vi "Res_stabiliz.vi"(4 "Точность ThRes":dbl step=0.01, 5 "Up_Volt_limit":dbl=5.0, 6 "Optimum ThRes":dbl format="%#_6f", 7 "Low_Volt_limit":dbl=1.0, 8 "TEC_Source":refnum<k15> caption="instrument handle", 9 "4070_address":refnum<k15>="PXI3Slot6_4 (1)" caption="4070_out", 10 "channel name":string, 11 "Start Voltage":dbl=3.0 format="%#.7f") -> (0 "Error message":string, 1 "Подстроенное напряжение":dbl, 2 "ThRes value":dbl, 3 "thRes_adj":dbl format="%0.2f")   [LabVIEW 2013]
uses:
  <instrlib>/niDMM/nidmm.llb/niDMM Resolution in Digits.ctl
  <instrlib>/niDMM/nidmm.llb/niDMM Function.ctl
  <vilib>/Analysis/baseanly.llb/Mean (DBL).vi
  <instrlib>/niDMM/nidmm.llb/niDMM Configure Measurement Digits.vi
  <vilib>/Analysis/NI_AALBase.lvlib
panel:
  out "Необходимая подстройка\nНапряжения":dbl
  out "Разница ThRes":dbl
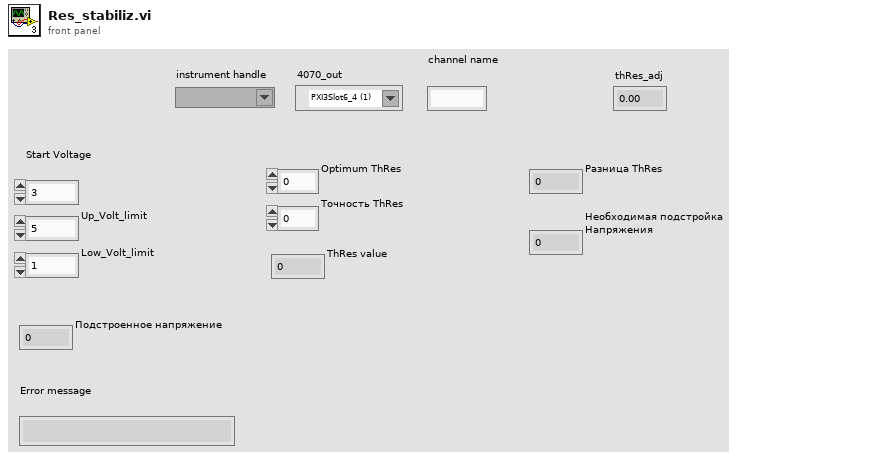
[diagram p1: front panel]
types:
  T1 = typedef "niDMM Function.ctl" = enum16{"DC Volts", "AC Volts", "DC Current", "AC Current", "2-wire Resistance", "4-wire Resistance", "Diode", "Frequency", "Period", "AC Volts DC Coupled", "Capacitance", "Inductance", "Temperature"}
  T2 = typedef "niDMM Resolution in Digits.ctl" = dbl
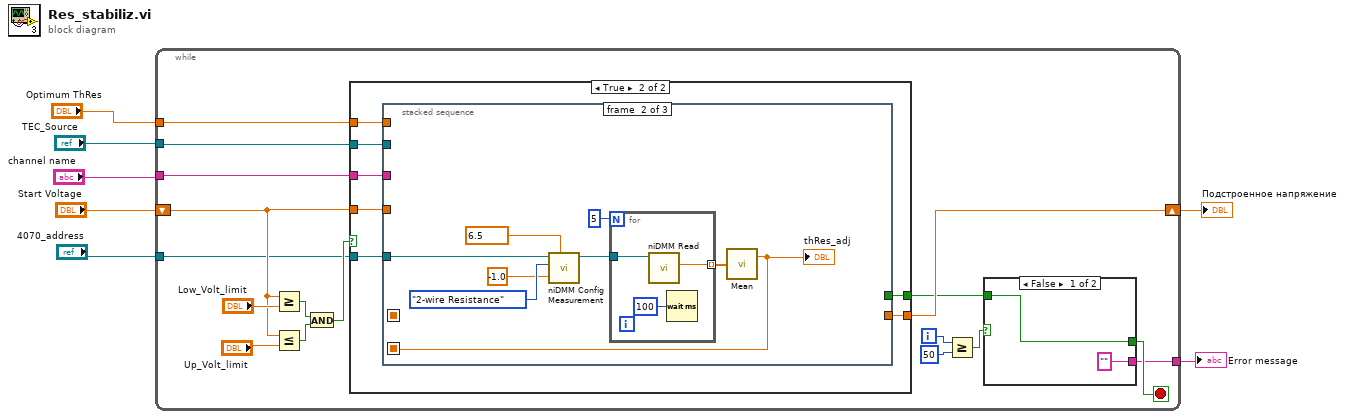
[diagram p0: block diagram]
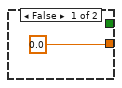
[diagram p2: hidden frame]
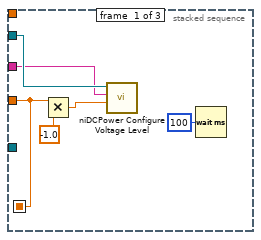
[diagram p3: hidden frame]
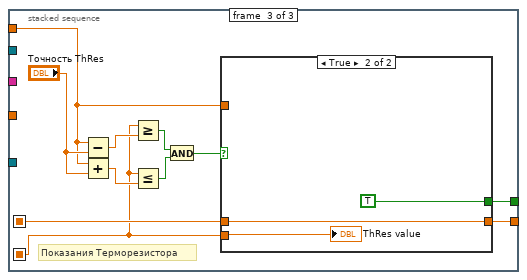
[diagram p4: hidden frame]
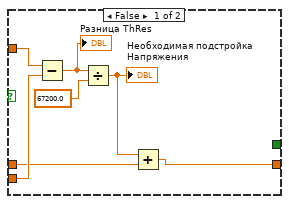
[diagram p5: hidden frame]
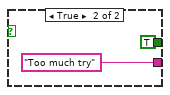
[diagram p6: hidden frame]
diagram:
  n1 = while {
    tunnel: "Optimum ThRes" -> [w12]
    tunnel: "channel name" -> [w13]
    tunnel: "TEC_Source" -> [w14]
    tunnel: "4070_address" -> [w11]
    shift-right: [w10] -> w4
    shift-left: "Start Voltage" -> [w15]
    tunnel: [w8] -> w3
    i -> [w21]
    stop <- w22 stop-if-true
    n2 = Greater Or Equal?(x=w15, y="Low_Volt_limit") -> (x >= y?=w20:bool)
    n3 = Less Or Equal?(x=w15, y="Up_Volt_limit") -> (x <= y?=w19:bool)
    n4 = And(x=w20, y=w19) -> (x .and. y?=w16:bool)
    n5 = case shown="True" w16 {
      tunnel: w15 -> [_ w30]
      tunnel: w14 -> [_ w32]
      tunnel: w13 -> [_ w31]
      tunnel: w12 -> [_ w28]
      tunnel: w11 -> [_ w29]
      tunnel: [0.0 w27] -> w10
      tunnel: [_ w26] -> w9
      frame False {
      }
      frame True {
        n6 = stacked-sequence {
          seq-local: [w33 _ _] -> [_ _ w54]
          seq-local: [_ w39 _] -> [_ _ w51]
          tunnel: w32 -> [w38 _ _]
          tunnel: w31 -> [w37 _ _]
          tunnel: w30 -> [w33 _ _]
          tunnel: w29 -> [_ w40 _]
          tunnel: w28 -> [_ _ w50]
          tunnel: [_ _ w53] -> w27
          tunnel: [_ _ w52] -> w26
          frame #0 {
            n7 = Multiply(x=w33, y=-1.0) -> (x*y=w34:dbl)
            n8 = call <instrlib>:"niDCPower Configure Voltage Level.vi"("voltage level"=w34, "channel name"=w37, "instrument handle"=w38) -> ()  [unwired: 7 in, 2 out]
            n9 = Wait (ms)(milliseconds to wait=u32 100) -> ()  [unwired: 1 out]
          }
          frame #1 {
            w43 = T2 6.5 items=["3 1/2"=3.5, "4 1/2"=4.5, "5 1/2"=5.5, "6 1/2"=6.5, "7 1/2"=7.5] ("Resolution in Digits")
            n10 = call-poly <instrlib>:"niDMM Config Measurement.vi"("Range"=-1.0 ("Configuration:Measurement Options:Max Frequency"), "Resolution in Digits"=w43, "Function"=niDMM_Function."2-wire Resistance" ("multimeter mode"), "instrument handle"=w40) -> ("instrument handle out"=w44:refnum<k15>)  [unwired: 6 in, 1 out]
            n11 = for {
              N: 5 -> [_]
              tunnel: w44 -> [w48]
              tunnel: [w47] -> w45 mode=indexing
              n12 = call <instrlib>:"niDMM Read.vi"("instrument handle"=w48) -> ("Measurement"=w47:dbl)  [unwired: 8 in, 2 out]
              n13 = Wait (ms)(milliseconds to wait=u32 100) -> ()  [unwired: 1 out]
            }
            n14 = call-poly <vilib>:"Mean.vi"("X"=w45) -> ("mean"=w39:dbl)  [unwired: 1 out]
            "thRes_adj" <- w39
          }
          frame #2 {
            # "Показания Терморезистора"
            n15 = Subtract(x=w50, y="Точность ThRes") -> (x-y=w58:dbl)
            n16 = Add(x=w50, y="Точность ThRes") -> (x+y=w59:dbl)
            n17 = Greater Or Equal?(x=w51, y=w58) -> (x >= y?=w60:bool)
            n18 = Less Or Equal?(x=w51, y=w59) -> (x <= y?=w56:bool)
            n19 = And(x=w60, y=w56) -> (x .and. y?=w55:bool)
            n20 = case shown="True" w55 {
              tunnel: [w61 w70] -> w53
              tunnel: w54 -> [w63 w70]
              tunnel: [_ TRUE] -> w52
              tunnel: w51 -> [w64 w68]
              tunnel: w50 -> [w65 _]
              frame False {
                n21 = Subtract(x=w65, y=w64) -> (x-y=w66:dbl)
                "Разница ThRes" <- w66
                n22 = Divide(x=w66, y=67200.0) -> (x/y=w62:dbl)
                "Необходимая подстройка\nНапряжения" <- w62
                n23 = Add(x=w62, y=w63) -> (x+y=w61:dbl)
              }
              frame True {
                "ThRes value" <- w68
              }
            }
          }
        }
      }
    }
    n24 = Greater Or Equal?(x=w21, y=50) -> (x >= y?=w23:bool)
    n25 = case shown="False" w23 {
      tunnel: ["" "Too much try"] -> w8
      tunnel: [w72 TRUE] -> w22
      tunnel: w9 -> [w72 _]
      frame False {
      }
      frame True {
      }
    }
  }
  "Подстроенное напряжение" <- w4
  "Error message" <- w3
